vi "Day06-01_수업.vi"   [LabVIEW 2021]
uses:
  <vilib>/DAQmx/create/channels.llb/DAQmx Create Channel (AI-Voltage-Basic).vi
  <vilib>/DAQmx/configure/timing.llb/DAQmx Timing (Sample Clock).vi
  <vilib>/DAQmx/read.llb/DAQmx Read (Analog 2D DBL NChan NSamp).vi
  <vilib>/DAQmx/write.llb/DAQmx Write (Analog 1D DBL NChan 1Samp).vi
panel:
  # "DAQ \n : 여러가지 물리적인 신호들을 데이터로 수집하는 것"
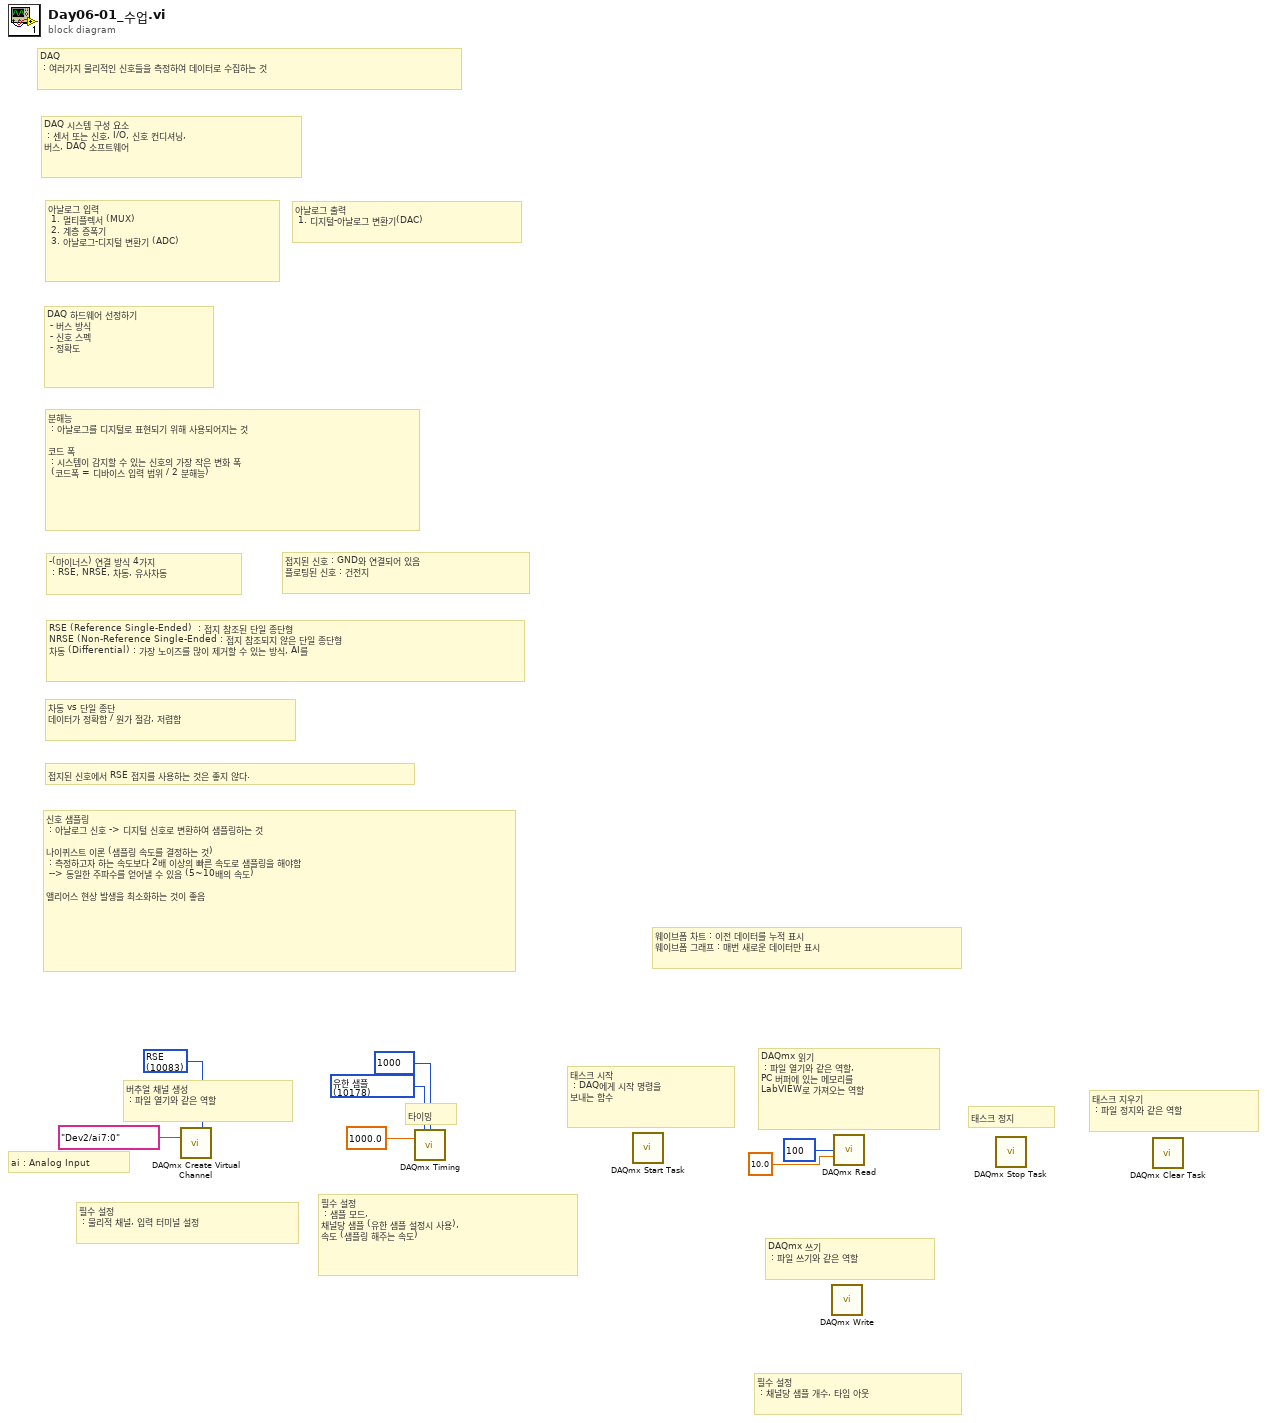
[diagram p0: block diagram]
diagram:
  w5 = 10178 items=["유한 샘플"=10178, "연속 샘플"=10123, "하드웨어 타이밍에 의한 단일 포인트"=12522] ("sample mode")
  w6 = 10083 items=["기본"=-1, "RSE"=10083, "NRSE"=10078, "차동"=10106, "유사 차동"=12529] ("input terminal configuration")
  # "태스크 지우기\n : 파일 정지와 같은 역할"
  # "태스크 정지"
  # "DAQmx 쓰기\n : 파일 쓰기와 같은 역할"
  # "필수 설정\n : 채널당 샘플 개수, 타임 아웃"
  # "웨이브폼 차트 : 이전 데이터를 누적 표시\n웨이브폼 그래프 : 매번 새로운 데이터만 표시"
  # "DAQmx 읽기\n : 파일 열기와 같은 역할, \nPC 버퍼에 있는 메모리를\nLabVIEW로 가져오는 역할"
  # "태스크 시작\n : DAQ에게 시작 명령을\n보내는 함수"
  # "타이밍"
  # "필수 설정\n : 샘플 모드, \n채널당 샘플 (유한 샘플 설정시 사용), \n속도 (샘플링 해주는 속도)"
  # "필수 설정\n : 물리적 채널, 입력 터미널 설정"
  # "ai : Analog Input"
  # "버추얼 채널 생성\n : 파일 열기와 같은 역할"
  # "신호 샘플링\n : 아날로그 신호 -> 디지털 신호로 변환하여 샘플링하는 것\n\n나이퀴스트 이론 (샘플링 속도를 결정하는 것)\n : 측정하고자 하는 속도보다 2배 이상의 빠른 속도로 샘플링을 해야함\n --> 동일한 주파수를 얻어낼 수 있음 (5~10배의 속도)\n\n앨리어스 현상 발생을 최소화하는 것이 좋음"
  # "접지된 신호에서 RSE 접지를 사용하는 것은 좋지 않다."
  # "차동 vs 단일 종단\n데이터가 정확함 / 원가 절감, 저렴함"
  # "RSE (Reference Single-Ended)  : 접지 참조된 단일 종단형\nNRSE (Non-Reference Single-Ended : 접지 참조되지 않은 단일 종단형\n차동 (Differential) : 가장 노이즈를 많이 제거할 수 있는 방식, AI를"
  # "접지된 신호 : GND와 연결되어 있음\n플로팅된 신호 : 건전지"
  # "-(마이너스) 연결 방식 4가지\n : RSE, NRSE, 차동, 유사차동"
  # "분해능\n : 아날로그를 디지털로 표현되기 위해 사용되어지는 것\n\n코드 폭\n : 시스템이 감지할 수 있는 신호의 가장 작은 변화 폭\n (코드폭 = 디바이스 입력 범위 / 2 분해능)"
  # "DAQ 하드웨어 선정하기\n - 버스 방식\n - 신호 스펙\n - 정확도"
  # "아날로그 출력\n 1. 디지털-아날로그 변환기(DAC)"
  # "아날로그 입력\n 1. 멀티플렉서 (MUX)\n 2. 계층 증폭기\n 3. 아날로그-디지털 변환기 (ADC)"
  # "DAQ 시스템 구성 요소\n : 센서 또는 신호, I/O, 신호 컨디셔닝, \n버스, DAQ 소프트웨어"
  # "DAQ \n : 여러가지 물리적인 신호들을 측정하여 데이터로 수집하는 것"
  n1 = call-poly <vilib>:"DAQmx Create Virtual Channel.vi"("input terminal configuration"=w6, "physical channels"=tag "Dev2/ai7:0") -> ()  [unwired: 12 in, 2 out]
  n2 = call-poly <vilib>:"DAQmx Timing.vi"("sample mode"=w5, "samples per channel"=1000, "rate"=1000.0) -> ()  [unwired: 11 in, 2 out]
  n3 = call <vilib>:"DAQmx Start Task.vi"() -> ()  [unwired: 14 in, 2 out]
  n4 = call-poly <vilib>:"DAQmx Write.vi"() -> ()  [unwired: 13 in, 3 out]
  n5 = call-poly <vilib>:"DAQmx Read.vi"("number of samples per channel"=100, "timeout"=10.0) -> ()  [unwired: 11 in, 3 out]
  n6 = call <vilib>:"DAQmx Stop Task.vi"() -> ()  [unwired: 14 in, 2 out]
  n7 = call <vilib>:"DAQmx Clear Task.vi"() -> ()  [unwired: 15 in, 1 out]
